vi "Set TEC SP.vi"(8 "error in":errorcluster, 10 "sp":sgl, 11 "CRDS in":refnum<class "CRDS.lvclass">) -> (0 "error out":errorcluster, 3 "CRDS out":refnum<class "CRDS.lvclass">)   [LabVIEW 2011, in "CRDS.lvclass"]
uses:
  CRDS.lvclass
  Reusable/Serial IO/TE Cooler/TE Cooler.lvclass
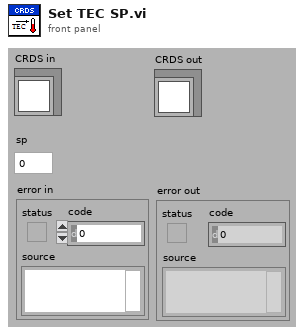
[diagram p1: front panel]
types:
  T1 = cluster{"YAG Ctr":refnum<k21>, "Diode Ctr":refnum<k21>, "Gated Ctr":refnum<k21>, "LF AI":refnum<k21>, "HF AI":refnum<k21>, "valveIn":refnum<k21>, "valveOut":refnum<k21>}
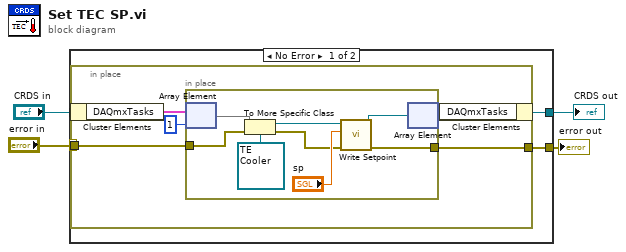
[diagram p0: block diagram]
diagram:
  n1 = case shown="No Error" "error in" {
    selector: "error in" -> [w7 w23]
    tunnel: [w5 w23] -> w3
    tunnel: [w6 w22] -> w1
    tunnel: "CRDS in" -> [w8 w22]
    frame No Error {
      n2 = in-place {
        in-place-border: w7 -> [w11]
        in-place-border: [w9] -> w5
        n3 = in-place-cluster #1(w8) -> ("DAQmxTasks"=w13:T1)
        n4 = in-place {
          in-place-border: w11 -> [w19]
          in-place-border: [w15] -> w9
          n5 = in-place-array #2(w13, 1) -> (w21)
          n6 = To More Specific Class(target class=refnum<class "TE Cooler.lvclass"> refnum ("TE Cooler.lvclass"), reference=w21, error in=w19) -> (specific class reference=w18:refnum<class "TE Cooler.lvclass">, error out=w16:errorcluster)
          n7 = call "Write Setpoint.vi"("error in"=w16, "SP"="sp", "TE Cooler in"=w18) -> ("error out"=w15:errorcluster, "TE Cooler out"=w14:refnum<class "TE Cooler.lvclass">)  [unwired: 7 in]
          n8 = in-place-array #2(w14) -> (w10)  [unwired: 1 out]
        }
        n9 = in-place-cluster #1("DAQmxTasks"=w10) -> (w6:refnum<class "CRDS.lvclass">)
      }
    }
    frame Error {
    }
  }
  "error out" <- w3
  "CRDS out" <- w1
